vi "JSONToPacket.vi"(8 "ErrorIn":errorcluster, 11 "JSONIn":refnum<class "JSON Value.lvclass">) -> (0 "ErrorOut":errorcluster, 2 "Packet":T1={"ID"=0, "SamplesNr"=0, "Samples"=[], "MeasurementConfig"={"Frequency"=100, "Resolution[b]"=4, "AccelFSRange"=enum."+/-2g", "GyroFSRange"=enum."+/-250dps"}, "Comment"=""} {"MeasurementConfig"."Resolution[b]" min=4 max=16 step=1; "MeasurementConfig"."Frequency" min=1 max=10000000 step=1}, 3 "JSONOut":refnum<class "JSON Value.lvclass">)   [LabVIEW 2016]
doc: "Convert JSON to Packet."
uses:
  FallSensor/Packet.ctl
  FallSensor/Sample.ctl
  FallSensor/Reading.ctl
  FallSensor/MeasurementConfig.ctl
  FallSensor/Measurement/AccelFSRange.ctl
  FallSensor/Measurement/GyroFSRange.ctl
  <vilib>/addons/JSON API/JSON Value/JSON Value.lvclass
  <vilib>/addons/JSON API/JSON Value/Get Object Item by Name.vi
  <vilib>/addons/JSON API/JSON Scalar/Get as U32.vi
  <vilib>/addons/JSON API/JSON Scalar/Get as Text.vi
  <vilib>/addons/JSON API/JSON Array/Get Array.vi
  <vilib>/addons/JSON API/Get Polymorphic/JSON GetSet.lvlib
  <vilib>/addons/JSON API/JSON Scalar/JSON Scalar.lvclass
  <vilib>/addons/JSON API/JSON Array/JSON Array.lvclass
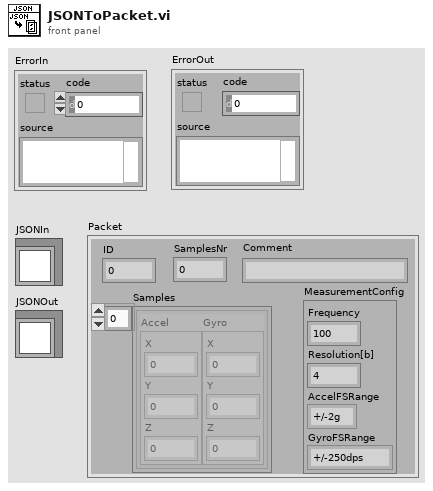
[diagram p1: front panel]
types:
  T1 = typedef "Packet.ctl" = cluster{"ID":u32, "SamplesNr":u32, "Samples":T2[], "MeasurementConfig":T4, "Comment":string}
  T2 = typedef "Sample.ctl" = cluster{"Accel":T3, "Gyro":T3}
  T3 = typedef "Reading.ctl" = cluster{"X":i16, "Y":i16, "Z":i16}
  T4 = typedef "MeasurementConfig.ctl" = cluster{"Frequency":u32, "Resolution[b]":u32, "AccelFSRange":T5, "GyroFSRange":T6}
  T5 = typedef "AccelFSRange.ctl" = enum16{"+/-2g", "+/-4g", "+/-8g", "+/-16g"}
  T6 = typedef "GyroFSRange.ctl" = enum16{"+/-250dps", "+/-500dps", "+/-1000dps", "+/-2000dps"}
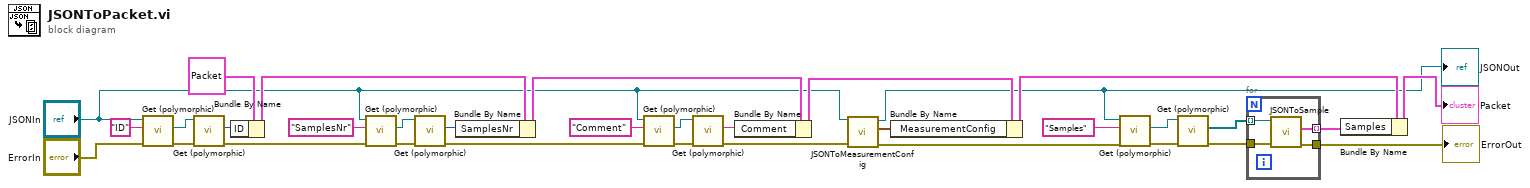
[diagram p0: block diagram]
diagram:
  n1 = call-poly <vilib>:"Get (polymorphic).vi"("error in (no error)"="ErrorIn", "name"="ID", "JSON Value In"="JSONIn") -> ("error out"=w32:errorcluster, "Value"=w26:refnum<class "JSON Value.lvclass">)  [unwired: 5 in, 2 out]
  n2 = call-poly <vilib>:"Get (polymorphic).vi"("error in (no error)"=w32, "JSON Scalar in"=w26) -> ("error out"=w24:errorcluster, "Number"=w31:u32)  [unwired: 7 in, 1 out]
  n3 = Bundle By Name(cluster=T1 {"ID"=0, "SamplesNr"=0, "Samples"=[], "MeasurementConfig"={"Frequency"=100, "Resolution[b]"=4, "AccelFSRange"=enum."+/-2g", "GyroFSRange"=enum."+/-250dps"}, "Comment"=""} ("Packet 2"), "ID"=w31) -> (w25:T1)
  n4 = call-poly <vilib>:"Get (polymorphic).vi"("error in (no error)"=w24, "name"="SamplesNr", "JSON Value In"="JSONIn") -> ("error out"=w28:errorcluster, "Value"=w8:refnum<class "JSON Value.lvclass">)  [unwired: 5 in, 2 out]
  n5 = call-poly <vilib>:"Get (polymorphic).vi"("error in (no error)"=w28, "JSON Scalar in"=w8) -> ("error out"=w7:errorcluster, "Number"=w29:u32)  [unwired: 7 in, 1 out]
  n6 = Bundle By Name(cluster=w25, "SamplesNr"=w29) -> (w6:T1)
  n7 = call-poly <vilib>:"Get (polymorphic).vi"("error in (no error)"=w7, "name"="Comment", "JSON Value In"="JSONIn") -> ("error out"=w10:errorcluster, "Value"=w12:refnum<class "JSON Value.lvclass">)  [unwired: 5 in, 2 out]
  n8 = call-poly <vilib>:"Get (polymorphic).vi"("error in (no error)"=w10, "JSON Scalar in"=w12) -> ("error out"=w4:errorcluster, "LabVIEW Text"=w9:string)  [unwired: 7 in, 1 out]
  n9 = Bundle By Name(cluster=w6, "Comment"=w9) -> (w5:T1)
  n10 = call "JSONToMeasurementConfig.vi"("ErrorIn"=w4, "JSONIn"="JSONIn") -> ("ErrorOut"=w21:errorcluster, "MeasurementConfig"=w23:T4, "JSONOut"=w1:refnum<class "JSON Value.lvclass">)  [unwired: 7 in]
  "JSONOut" <- w1
  n11 = Bundle By Name(cluster=w5, "MeasurementConfig"=w23) -> (w14:T1)
  n12 = call-poly <vilib>:"Get (polymorphic).vi"("error in (no error)"=w21, "name"="Samples", "JSON Value In"=w1) -> ("error out"=w20:errorcluster, "Value"=w19:refnum<class "JSON Value.lvclass">)  [unwired: 5 in, 2 out]
  n13 = call-poly <vilib>:"Get (polymorphic).vi"("error in (no error)"=w20, "JSON Array in"=w19) -> ("error out"=w18:errorcluster, "Array"=w16:refnum<class "JSON Value.lvclass">[])  [unwired: 7 in, 1 out]
  n14 = for {
    tunnel: w18 -> [w37]
    tunnel: [w36] -> w17
    tunnel: w16 -> [w35] mode=indexing
    tunnel: [w34] -> w15 mode=indexing
    n15 = call "JSONToSample.vi"("ErrorIn"=w37, "JSONIn"=w35) -> ("ErrorOut"=w36:errorcluster, "Sample"=w34:T2)  [unwired: 7 in, 1 out]
  }
  "ErrorOut" <- w17
  n16 = Bundle By Name(cluster=w14, "Samples"=w15) -> (→"Packet":T1)
